vi "Set Compiler Level.vi"(8 "error in (no error)":errorcluster, 10 "compiler Level (1)":u32=1, 11 "NI_AB_API_Build in":refnum<class "NI_AB_API_Build.lvclass">) -> (0 "error out":errorcluster, 3 "NI_AB_API_Build out":refnum<class "NI_AB_API_Build.lvclass">)   [LabVIEW 2020, in "NI_AB_API_Build.lvclass"]
uses:
  <vilib>/AppBuilder/AB_API/Build/NI_AB_API_Build.lvclass
  <vilib>/AppBuilder/AB_API/Build/NI_AB_API_Build.lvclass/NI_AB_API_Build.ctl
panel:
  # "0: SSE2 optimization disabled\n1: SSE2 optimization enabled"
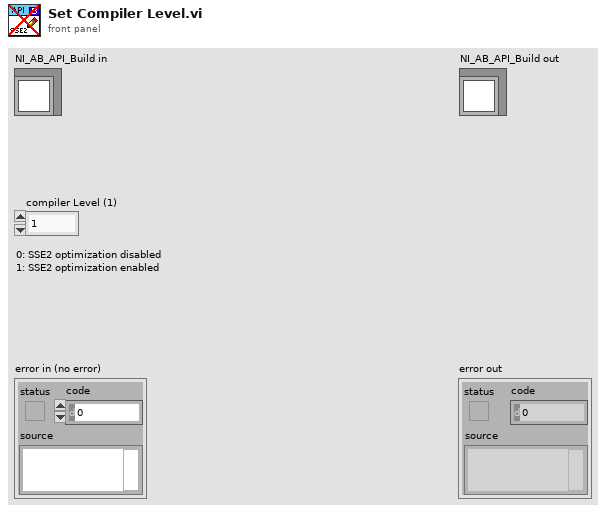
[diagram p1: front panel]
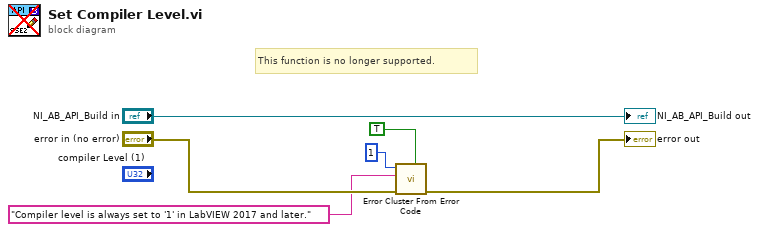
[diagram p0: block diagram]
diagram:
  # "This function is no longer supported."
  n1 = call <vilib>:"Error Cluster From Error Code.vi"("is warning? (False)"=TRUE, "error in (no error)"="error in (no error)", "error message (\"\")"="Compiler level is always set to '1' in LabVIEW 2017 and later." ("error message (\"\")"), "error code (0)"=1) -> ("error out"=→"error out":errorcluster)  [unwired: 5 in]
  "NI_AB_API_Build out" <- "NI_AB_API_Build in"
